vi "StandardMethodsForSetGetControlValues.vi"() -> ()   [LabVIEW 2019]
panel:
  in  "VI Name 2":string
  in  "Values to Set":variant[](array[variant])
  out "Read Values":variant[](array[variant])
  in  "Control Names":string[](array[string])
  out "Read Value":variant
  in  "Value to Set":variant
  in  "Control Name":string
  in  "VI Name":string
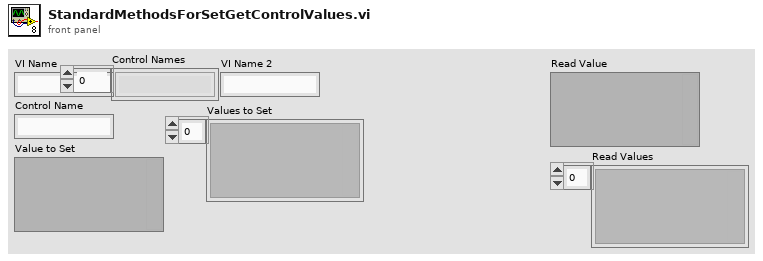
[diagram p1: front panel]
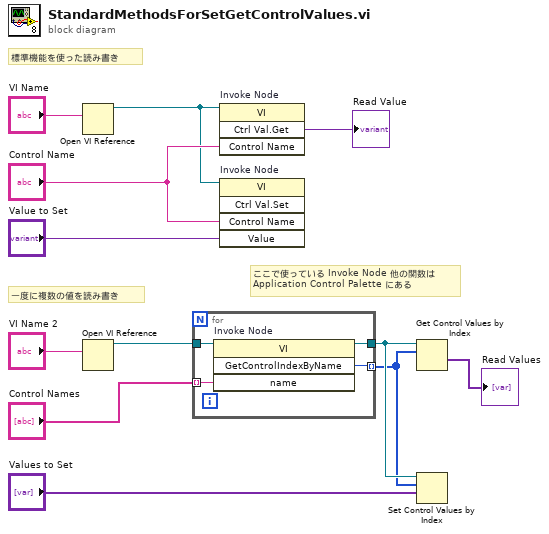
[diagram p0: block diagram]
diagram:
  # "ここで使っている Invoke Node 他の関数は \nApplication Control Palette にある"
  # "一度に複数の値を読み書き"
  # "標準機能を使った読み書き"
  n1 = Open VI Reference(vi path="VI Name") -> (vi reference=w8:refnum<vi>)  [unwired: 5 in, 1 out]
  n2 = Open VI Reference(vi path="VI Name 2") -> (vi reference=w7:refnum<vi>)  [unwired: 5 in, 1 out]
  n3 = for {
    tunnel: w7 -> [w16]
    tunnel: "Control Names" -> [w15] mode=indexing
    tunnel: [w14] -> w3 mode=indexing
    tunnel: [w13] -> w4
    n4 = invoke on="Invoke Node" class="VI" method="GetControlIndexByName"(reference=w16, "name"=w15) -> (reference out=w13:refnum<vi>, "GetControlIndexByName"=w14:i32)  [unwired: 2 in, 2 out]
  }
  n5 = invoke on="Invoke Node" class="VI" method="Ctrl Val.Get"(reference=w8, "Control Name"="Control Name") -> ("Get Control Value Variant"=→"Read Value":variant)  [unwired: 2 in, 3 out]
  n6 = invoke on="Invoke Node" class="VI" method="Ctrl Val.Set"(reference=w8, "Control Name"="Control Name", "Value"="Value to Set") -> ()  [unwired: 2 in, 5 out]
  n7 = Get Control Values by Index(0:w4, 1:w3) -> (10:→"Read Values":variant[])  [unwired: 1 in, 1 out]
  n8 = Set Control Values by Index(0:w4, 1:w3, 2:"Values to Set") -> ()  [unwired: 1 in, 1 out]
